vi "Start Logic.vi"(8 "error in":errorcluster, 9 "index (row)":i32, 10 "array":string[][](array[string]), 11 "Modbus master in":refnum<class "Modbus Master.lvclass">) -> (0 "error out":errorcluster, 3 "Modbus master out":refnum<class "Modbus Master.lvclass">, 4 "Time":string, 5 "Direction":string, 6 "Temp":string, 7 "Speed":string)   [LabVIEW 2014, in "Main Libraryv2.lvlib"]
uses:
  Control/Main Libraryv2.lvlib
  <vilib>/NI/Modbus Library/API/Master/Modbus Master.lvclass
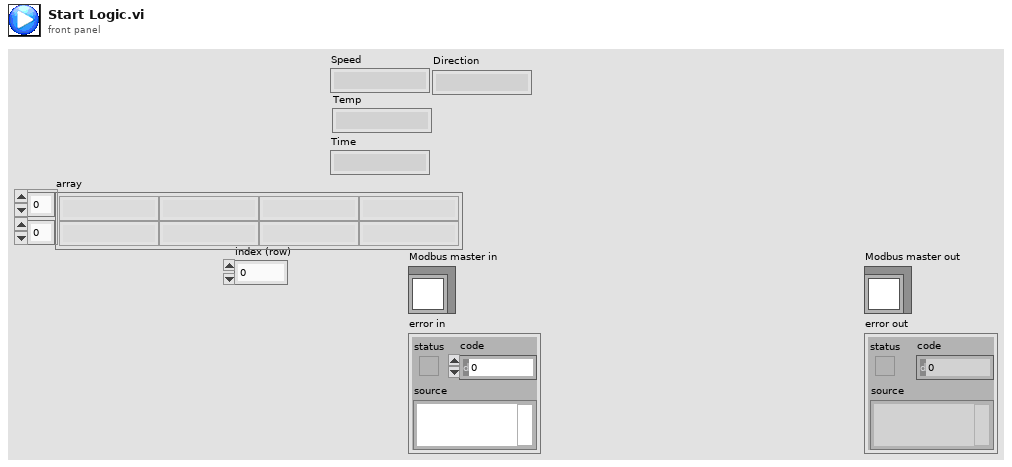
[diagram p1: front panel]
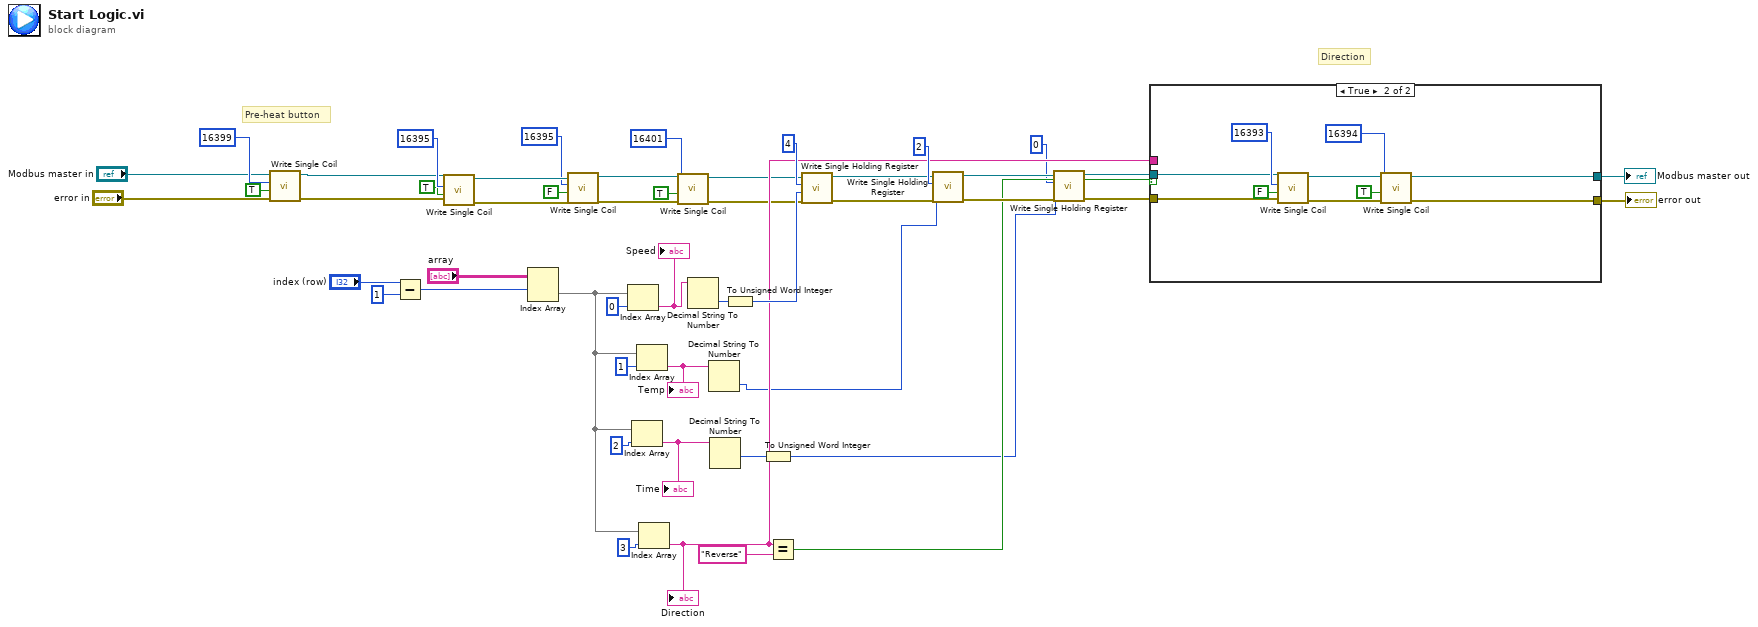
[diagram p0: block diagram]
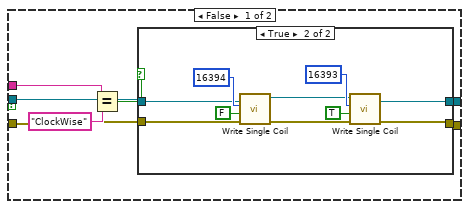
[diagram p2: hidden frame]
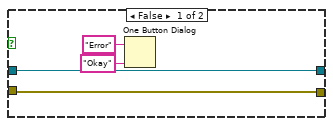
[diagram p3: hidden frame]
diagram:
  # "Direction"
  # "Pre-heat button"
  n1 = call-dynamic "Write Single Coil.vi"("error in"="error in", "coil to write"=TRUE, "address"=u16 16399, "Modbus master in"="Modbus master in") -> ("error out"=w42:errorcluster, "Modbus master out"=w44:refnum<class "Modbus Master.lvclass">)  [unwired: 6 in]
  n2 = Subtract(x="index (row)", y=1) -> (x-y=w22:i32)
  n3 = call-dynamic "Write Single Coil.vi"("error in"=w42, "coil to write"=TRUE, "address"=u16 16395, "Modbus master in"=w44) -> ("error out"=w41:errorcluster, "Modbus master out"=w43:refnum<class "Modbus Master.lvclass">)  [unwired: 6 in]
  n4 = Index Array(array="array", index (row)=w22) -> (element=w18:string[])  [unwired: 1 in]
  n5 = call-dynamic "Write Single Coil.vi"("error in"=w41, "coil to write"=FALSE, "address"=u16 16395, "Modbus master in"=w43) -> ("error out"=w4:errorcluster, "Modbus master out"=w7:refnum<class "Modbus Master.lvclass">)  [unwired: 6 in]
  n6 = Index Array(array=w18, index=0) -> (element=w32:string)
  "Speed" <- w32
  n7 = Index Array(array=w18, index=2) -> (element=w30:string)
  "Time" <- w30
  n8 = Index Array(array=w18, index=1) -> (element=w31:string)
  "Temp" <- w31
  n9 = Index Array(array=w18, index=3) -> (element=w15:string)
  "Direction" <- w15
  n10 = call-dynamic "Write Single Coil.vi"("error in"=w4, "coil to write"=TRUE, "address"=u16 16401, "Modbus master in"=w7) -> ("error out"=w5:errorcluster, "Modbus master out"=w6:refnum<class "Modbus Master.lvclass">)  [unwired: 6 in]
  n11 = Decimal String To Number(string=w32) -> (number=w27:i32)  [unwired: 2 in, 1 out]
  n12 = Decimal String To Number(string=w31) -> (number=w10:i32)  [unwired: 2 in, 1 out]
  n13 = Decimal String To Number(string=w30) -> (number=w25:i32)  [unwired: 2 in, 1 out]
  n14 = To Unsigned Word Integer(number=w27) -> (unsigned 16bit integer=w26:u16)
  n15 = To Unsigned Word Integer(number=w25) -> (unsigned 16bit integer=w9:u16)
  n16 = Equal?(x=w15, y="Reverse") -> (x = y?=w17:bool)
  n17 = call-dynamic "Write Single Holding Register.vi"("error in"=w5, "register to write"=w26, "address"=u16 4, "Modbus master in"=w6) -> ("error out"=w37:errorcluster, "Modbus master out"=w38:refnum<class "Modbus Master.lvclass">)  [unwired: 6 in]
  n18 = call-dynamic "Write Single Holding Register.vi"("error in"=w37, "register to write"=w10, "address"=u16 2, "Modbus master in"=w38) -> ("error out"=w35:errorcluster, "Modbus master out"=w36:refnum<class "Modbus Master.lvclass">)  [unwired: 6 in]
  n19 = call-dynamic "Write Single Holding Register.vi"("error in"=w35, "register to write"=w9, "address"=u16 0, "Modbus master in"=w36) -> ("error out"=w13:errorcluster, "Modbus master out"=w14:refnum<class "Modbus Master.lvclass">)  [unwired: 6 in]
  n20 = case shown="True" w17 {
    tunnel: w15 -> [w54 _]
    tunnel: w14 -> [w53 w75]
    tunnel: w13 -> [w52 w74]
    tunnel: [w50 w73] -> w12
    tunnel: [w51 w72] -> w11
    frame False {
      n21 = Equal?(x=w54, y="ClockWise") -> (x = y?=w56:bool)
      n22 = case shown="True" w56 {
        tunnel: w53 -> [w60 w65]
        tunnel: w52 -> [w59 w64]
        tunnel: [w59 w63] -> w51
        tunnel: [w60 w62] -> w50
        frame False {
          n23 = One Button Dialog(message="Error", button name ("OK")="Okay") -> ()  [unwired: 1 out]
        }
        frame True {
          n24 = call-dynamic "Write Single Coil.vi"("error in"=w64, "coil to write"=FALSE, "address"=u16 16394, "Modbus master in"=w65) -> ("error out"=w68:errorcluster, "Modbus master out"=w69:refnum<class "Modbus Master.lvclass">)  [unwired: 6 in]
          n25 = call-dynamic "Write Single Coil.vi"("error in"=w68, "coil to write"=TRUE, "address"=u16 16393, "Modbus master in"=w69) -> ("error out"=w63:errorcluster, "Modbus master out"=w62:refnum<class "Modbus Master.lvclass">)  [unwired: 6 in]
        }
      }
    }
    frame True {
      n26 = call-dynamic "Write Single Coil.vi"("error in"=w74, "coil to write"=FALSE, "address"=u16 16393, "Modbus master in"=w75) -> ("error out"=w78:errorcluster, "Modbus master out"=w79:refnum<class "Modbus Master.lvclass">)  [unwired: 6 in]
      n27 = call-dynamic "Write Single Coil.vi"("error in"=w78, "coil to write"=TRUE, "address"=u16 16394, "Modbus master in"=w79) -> ("error out"=w72:errorcluster, "Modbus master out"=w73:refnum<class "Modbus Master.lvclass">)  [unwired: 6 in]
    }
  }
  "Modbus master out" <- w12
  "error out" <- w11
